vi "Play sound start trial.vi"(10 "LED Voltage":dbl, 11 "Bright/mixed mode \nLED voltage (V)":dbl) -> ()   [LabVIEW 2013]
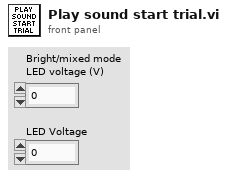
[diagram p1: front panel]
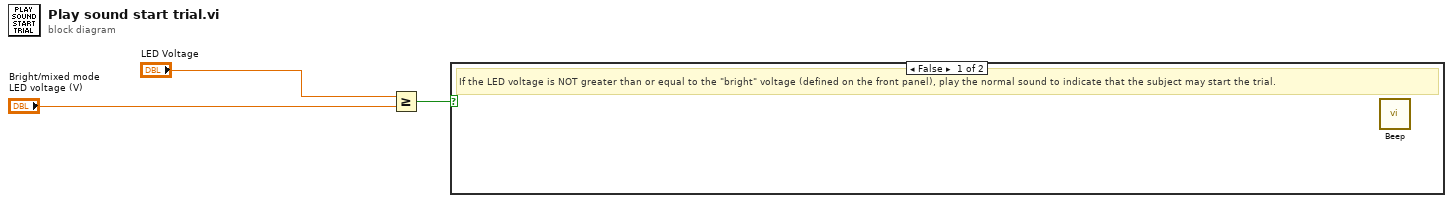
[diagram p0: block diagram]
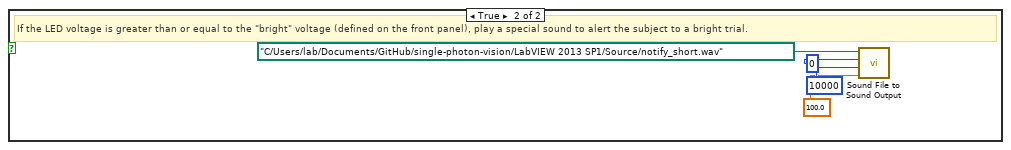
[diagram p2: hidden frame]
diagram:
  n1 = Greater Or Equal?(x="LED Voltage", y="Bright/mixed mode \nLED voltage (V)") -> (x >= y?=w3:bool)
  n2 = case shown="False" w3 {
    frame False {
      # "If the LED voltage is NOT greater than or equal to the \"bright\" voltage (defined on the front panel), play the normal sound to indicate that the subject may start the trial."
      n3 = call <vilib>:"Beep.vi"() -> ()  [unwired: 12 in]
    }
    frame True {
      # "If the LED voltage is greater than or equal to the \"bright\" voltage (defined on the front panel), play a special sound to alert the subject to a bright trial."
      n4 = call "Sound File to Sound Output.vi"("Volume"=100.0, "Number of Samples/Iteration"=10000, "Device ID"=u32 0, "File Path"=path "C:/Users/lab/Documents/GitHub/single-photon-vision/LabVIEW 2013 SP1/Source/notify_short.wav") -> ()
    }
  }
